vi "getEventSummaryState.vi"(11 "Publisher in":refnum<class "Publisher.lvclass">) -> (2 "EventSummaryState":T1, 3 "Publisher out":refnum<class "Publisher.lvclass">)   [LabVIEW 2016, in "Publisher.lvclass"]
uses:
  Publisher.lvclass
  DataTypes/Topics/EventSummaryState.ctl
  DataTypes/Topics/Parts/Timestamp.ctl
  DataTypes/Topics/Parts/SummaryStates.ctl
  Publisher.lvclass/Publisher.ctl
  DataTypes/Topics/M1M3SupportTopics.lvlib
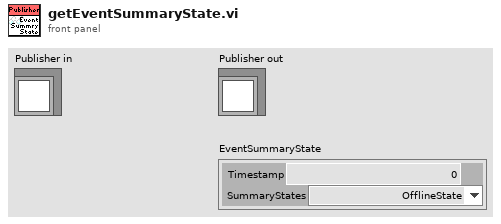
[diagram p1: front panel]
types:
  T1 = typedef "M1M3SupportTopics.lvlib/EventSummaryState.ctl" = cluster{"Timestamp":T2, "SummaryStates":T3}
  T2 = typedef "M1M3SupportTopics.lvlib/Timestamp.ctl" = dbl
  T3 = typedef "M1M3SupportTopics.lvlib/SummaryStates.ctl" = enum16{"OfflineState", "StandbyState", "DisabledState", "EnabledState", "FaultState"}
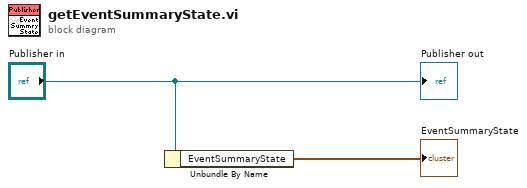
[diagram p0: block diagram]
diagram:
  n1 = Unbundle By Name("Publisher in") -> ("EventSummaryState"=→"EventSummaryState":T1)
  "Publisher out" <- "Publisher in"
